vi "Query Probe Model Number.vi"(0 "VISA resource name":refnum<visa-resource-name>, 5 "Channel Name (Channel 1)":i32(ring) items=["Channel 1", "Channel 2", "Channel 3", "Channel 4"], 11 "error in (no error)":errorcluster) -> (4 "VISA resource name out":refnum<visa-resource-name>, 6 "Probe Model Number":string, 15 "error out":errorcluster)   [LabVIEW 2016, in "Agilent 2000 3000 X-Series.lvlib"]
doc: "Returns the model number of a probe."
uses:
  Agilent 2000 3000 X-Series.lvlib
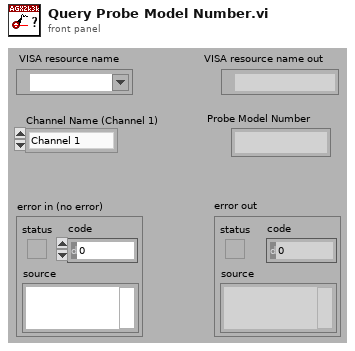
[diagram p1: front panel]
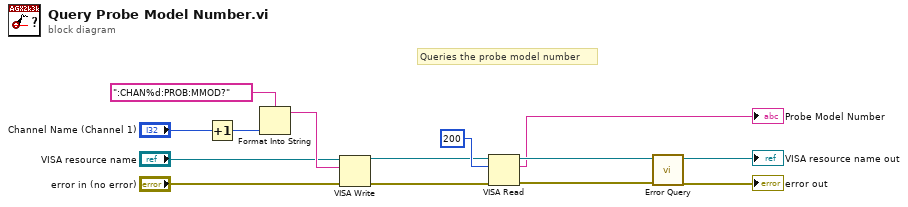
[diagram p0: block diagram]
diagram:
  # "Queries the probe model number"
  n1 = Increment(x="Channel Name (Channel 1)") -> (x+1=w3:i32)
  n2 = Format Into String(format string=":CHAN%d:PROB:MMOD?", w3) -> (resulting string=w5:string)  [unwired: 2 in, 1 out]
  n3 = VISA Write(VISA resource name="VISA resource name", write buffer=w5, error in (no error)="error in (no error)") -> (VISA resource name out=w10:refnum<visa-resource-name>, error out=w9:errorcluster)  [unwired: 1 out]
  n4 = VISA Read(VISA resource name=w10, byte count=u32 200, error in (no error)=w9) -> (VISA resource name out=w8:refnum<visa-resource-name>, read buffer=→"Probe Model Number":string, error out=w7:errorcluster)  [unwired: 1 out]
  n5 = call "Error Query.vi"("error in (no error)"=w7, "VISA resource name"=w8) -> ("error out"=→"error out":errorcluster, "VISA resource name out"=→"VISA resource name out":refnum<visa-resource-name>)  [unwired: 8 out]
